vi "Transition State.vi"(8 "Error In":errorcluster, 10 "Inputs":T1, 11 "Present  State":T2) -> (0 "Error Out":errorcluster, 3 "Next State":T2)   [LabVIEW 2018]
doc: "This VI uses the present state and inputs to determine the next state."
uses:
  controls/Enum Defining FSM State.ctl
  controls/Cluster for displaying  ABR switch states.ctl
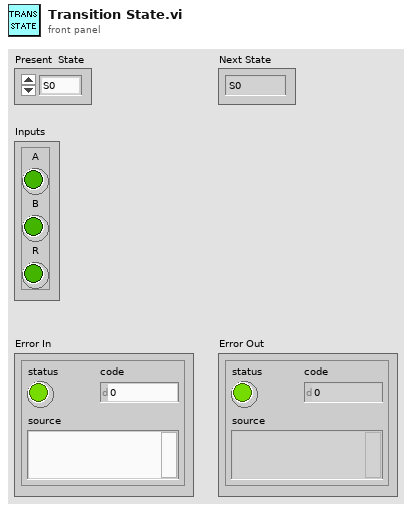
[diagram p1: front panel]
types:
  T1 = typedef "Cluster for displaying  ABR switch states.ctl" = cluster{"A":bool, "B":bool, "R":bool}
  T2 = typedef "Enum Defining FSM State.ctl" = enum16{"S0", "S1", "S2", "S3"}
  T3 = typedef "Enum Defining AB State.ctl" = enum16{"!A !B", "!A  B", " A !B", " A B"}
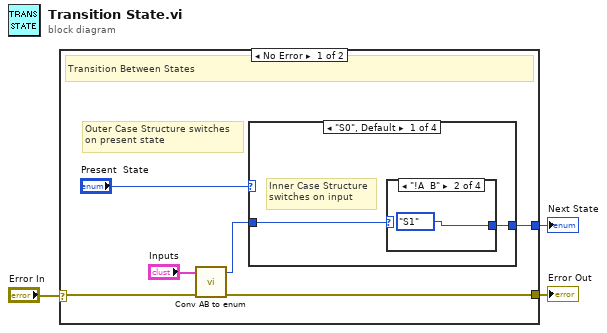
[diagram p0: block diagram]
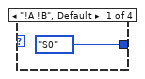
[diagram p2: hidden frame]
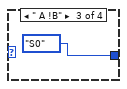
[diagram p3: hidden frame]
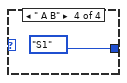
[diagram p4: hidden frame]
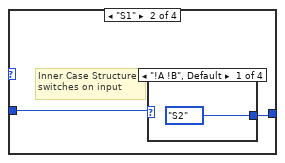
[diagram p5: hidden frame]
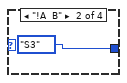
[diagram p6: hidden frame]
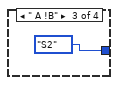
[diagram p7: hidden frame]
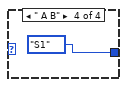
[diagram p8: hidden frame]
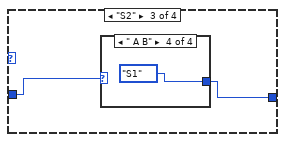
[diagram p9: hidden frame]
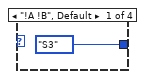
[diagram p10: hidden frame]
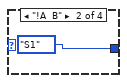
[diagram p11: hidden frame]
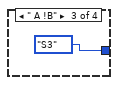
[diagram p12: hidden frame]
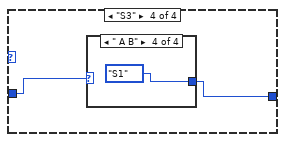
[diagram p13: hidden frame]
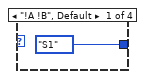
[diagram p14: hidden frame]
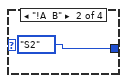
[diagram p15: hidden frame]
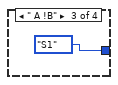
[diagram p16: hidden frame]
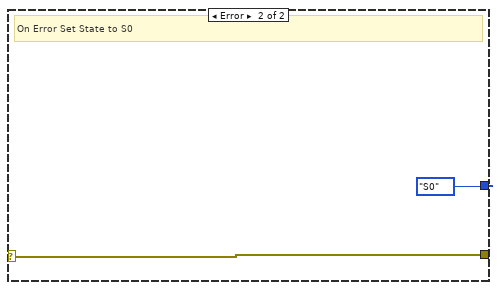
[diagram p17: hidden frame]
diagram:
  n1 = case shown="No Error" "Error In" {
    selector: "Error In" -> [w7 w35]
    tunnel: [w6 w35] -> w2
    tunnel: [w8 Enum_Defining_FSM_State."S0" ("State Enum")] -> w1
    frame No Error {
      # "Outer Case Structure switches\non present state"
      # "Transition Between States"
      n2 = call "Conv AB to enum.vi"("Error In"=w7, "Inputs"="Inputs") -> ("Error Out"=w6:errorcluster, "Input State"=w4:T3)  [unwired: 8 in]
      n3 = case shown="\"S0\", Default" "Present  State" {
        tunnel: [w11 w16 w23 w29] -> w8
        tunnel: w4 -> [w10 w17 w22 w28]
        frame "S0", Default {
          # "Inner Case Structure\nswitches on input"
          n4 = case shown="\"!A  B\"" w10 {
            tunnel: [Enum_Defining_FSM_State."S0" ("State Enum") Enum_Defining_FSM_State."S1" ("State Enum") Enum_Defining_FSM_State."S0" ("State Enum") Enum_Defining_FSM_State."S1" ("State Enum")] -> w11
            frame "!A !B", Default {
            }
            frame "!A  B" {
            }
            frame " A !B" {
            }
            frame " A B" {
            }
          }
        }
        frame "S1" {
          # "Inner Case Structure\nswitches on input"
          n5 = case shown="\"!A !B\", Default" w17 {
            tunnel: [Enum_Defining_FSM_State."S2" ("State Enum") Enum_Defining_FSM_State."S3" ("State Enum") Enum_Defining_FSM_State."S2" ("State Enum") Enum_Defining_FSM_State."S1" ("State Enum")] -> w16
            frame "!A !B", Default {
            }
            frame "!A  B" {
            }
            frame " A !B" {
            }
            frame " A B" {
            }
          }
        }
        frame "S2" {
          n6 = case shown="\" A B\"" w22 {
            tunnel: [Enum_Defining_FSM_State."S3" ("State Enum") Enum_Defining_FSM_State."S1" ("State Enum") Enum_Defining_FSM_State."S3" ("State Enum") Enum_Defining_FSM_State."S1" ("State Enum")] -> w23
            frame "!A !B", Default {
            }
            frame "!A  B" {
            }
            frame " A !B" {
            }
            frame " A B" {
            }
          }
        }
        frame "S3" {
          n7 = case shown="\" A B\"" w28 {
            tunnel: [Enum_Defining_FSM_State."S1" ("State Enum") Enum_Defining_FSM_State."S2" ("State Enum") Enum_Defining_FSM_State."S1" ("State Enum") Enum_Defining_FSM_State."S1" ("State Enum")] -> w29
            frame "!A !B", Default {
            }
            frame "!A  B" {
            }
            frame " A !B" {
            }
            frame " A B" {
            }
          }
        }
      }
    }
    frame Error {
      # "On Error Set State to S0"
    }
  }
  "Error Out" <- w2
  "Next State" <- w1
